vi "AMS Gas cRIO Outer Core.vi"() -> ()   [LabVIEW 2015]
uses:
  Actors/cRIO-CO2/Debugger.ctl
  Actors/cRIO-CO2 Messages/Assign Debugger to Actor Msg/Assign Debugger to Actor Msg.lvclass/Assign Debugger to Actor Msg.ctl
  <vilib>/ActorFramework/Message Enqueuer/Message Enqueuer.lvclass/Message Enqueuer.ctl
  Actors/cRIO-CO2 Messages/Unregister Actor Msg/Unregister Actor Msg.lvclass/Unregister Actor Msg.ctl
  <vilib>/ActorFramework/Message Enqueuer/Enqueue.vi
  <vilib>/ActorFramework/Message Priority Queue/Priority Enqueue.vi
  Actors/cRIO-CO2 Messages/Assign Debugger to Actor Msg/Assign Debugger to Actor Msg.lvclass
  Actors/cRIO-CO2 Messages/Stop All Actors Msg/Stop All Actors Msg.lvclass
  Actors/cRIO-CO2 Messages/Unregister Actor Msg/Unregister Actor Msg.lvclass
  <vilib>/NI_Real-Time Target Support.lvlib
  Actors/cRIO-CO2/cRIO-CO2.lvclass
  <resource>/objmgr/nisysapi.rc
panel:
  out "error out":errorcluster
  in  "Debug":u16(ring)
  out "Debugger Graph Chart":T1(graph)
  in  "Log":i32(listbox)
  out "Thermocouples":T2(graph)
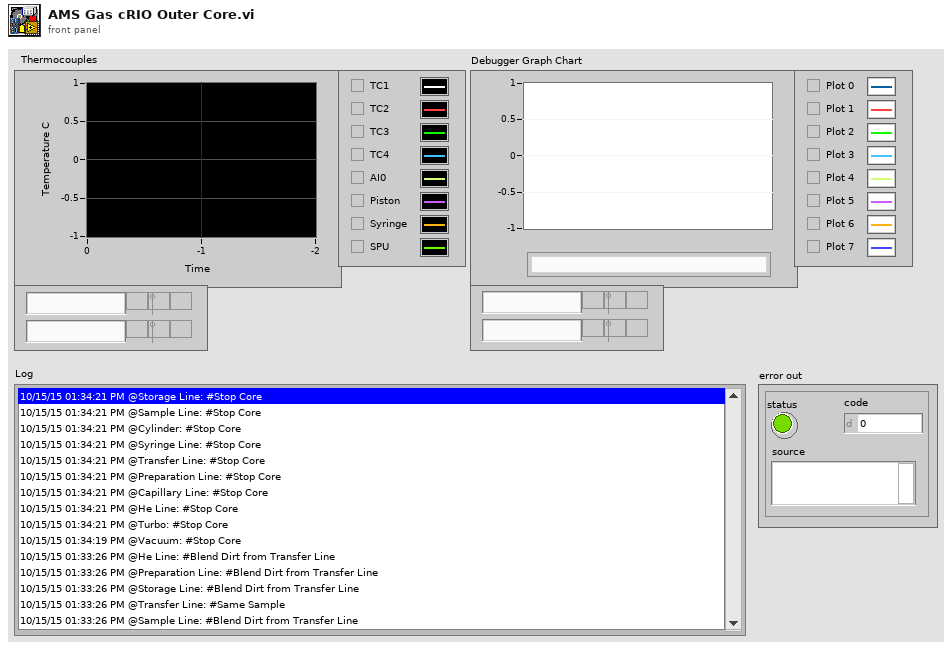
[diagram p1: front panel]
types:
  T1 = cluster{"dT/dt-Lower":dbl, "dT/dt":dbl, "dT/dt 2":dbl, "dT/dt 3":dbl, "dT/dt 4":dbl, "dT/dt-Lower 2":dbl, "dT/dt-Lower 3":dbl, "dT/dt 5":dbl}
  T2 = cluster{dbl, dbl, dbl, dbl, dbl, dbl, dbl, "Total (%)":dbl}
  T3 = cluster{"Numeric 0":dbl, "Numeric 1":dbl, "Numeric 2":dbl, "Numeric 3":dbl, "Numeric 4":dbl, "Numeric 5":dbl, "Numeric 6":dbl, "Numeric 7":dbl}
  T4 = typedef "cRIO-Carbondioxide.lvlib/cRIO-CO2.lvlib/cRIO-CO2.lvclass/Debugger.ctl" = cluster{"Log Ref":refnum<vi>, "Debugger Graph Chart Ref":refnum<vi>, "Debug Rng Ref":refnum<vi>}
  T5 = typedef "NI_Real-Time Target Support.lvlib/RT CPU Load.ctl" = cluster{"Total (%)":dbl, "Time Critical (%)":dbl, "Timed Structures (%)":dbl, "High (%)":dbl, "Above Normal (%)":dbl, "Normal (%)":dbl, "Background (%)":dbl, "Idle (%)":dbl, "ISR (%)":dbl}
  T6 = cluster{"Double":dbl, dbl, dbl, dbl, dbl, dbl, dbl, "Total (%)":dbl}
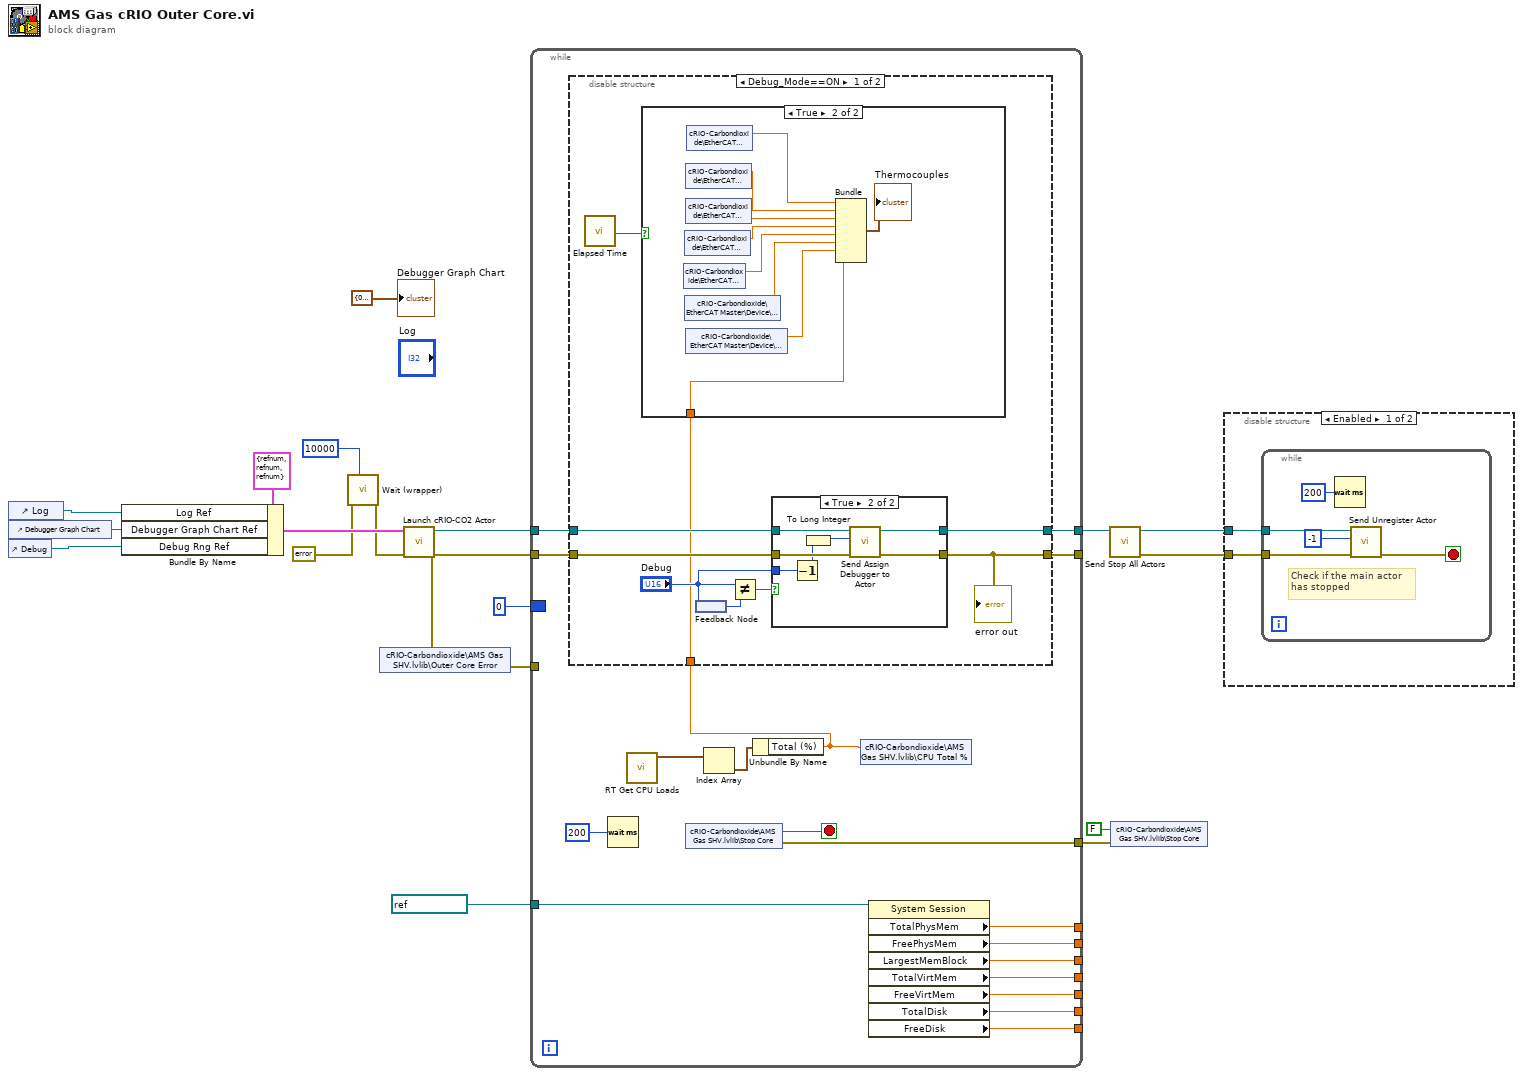
[diagram p0: block diagram]
diagram:
  n1 = control-ref of="Log"() -> (w8:refnum<vi>)
  n2 = control-ref of="Debugger Graph Chart"() -> (w6:refnum<vi>)
  n3 = control-ref of="Debug"() -> (w7:refnum<vi>)
  n4 = Bundle By Name(cluster=T4 {"Log Ref"=refnum, "Debugger Graph Chart Ref"=refnum, "Debug Rng Ref"=refnum} ("Refs for Debuging"), "Log Ref"=w8, "Debugger Graph Chart Ref"=w6, "Debug Rng Ref"=w7) -> (w17:T4)
  n5 = call "Wait (wrapper).vi"("milliseconds to wait (200)"=u32 10000, "error in (no error)"=errorcluster {"status"=FALSE, "code"=0, "source"=""}) -> ("error out"=w4:errorcluster)  [unwired: 9 in]
  n6 = call "Launch cRIO-CO2 Actor.vi"("error in (no error)"=w4, "Refs for Debuging"=w17) -> ("error out"=w11:errorcluster, "Caller-To-Actor Enqueuer"=w19:refnum<class "Message Enqueuer.lvclass">)  [unwired: 8 in]
  n7 = shared-variable "cRIO-Carbondioxide\\AMS Gas SHV.lvlib\\Outer Core Error"(w11) -> (error out=w2:errorcluster)  [unwired: 1 in]
  n8 = while {
    tunnel: w19 -> [w33]
    tunnel: w11 -> [w37]
    tunnel: [w36] -> w16
    border: u16 0 ("Debug") -> [_]
    tunnel: [w35] -> _
    tunnel: [w31] -> w10
    tunnel: w2 -> [_]
    tunnel: refnum<k21> "localhost" ("System Configuration") -> [w27]
    tunnel: [w26] -> _
    tunnel: [w25] -> _
    tunnel: [w24] -> _
    tunnel: [w23] -> _
    tunnel: [w22] -> _
    tunnel: [w21] -> _
    tunnel: [w20] -> _
    stop <- w32 stop-if-true
    n9 = Wait (ms)(milliseconds to wait=u32 200) -> ()  [unwired: 1 out]
    n10 = call <vilib>:"RT Get CPU Loads.vi"() -> ("CPU loads"=w29:T5[])  [unwired: 10 in, 1 out]
    n11 = shared-variable "cRIO-Carbondioxide\\AMS Gas SHV.lvlib\\Stop Core"() -> (w32:bool, error out=w31:errorcluster)  [unwired: 1 in]
    n12 = Index Array(array=w29) -> (element=w30:T5)  [unwired: 1 in]
    n13 = Unbundle By Name(w30) -> ("Total (%)"=w28:dbl)
    n14 = disable-structure shown="Debug_Mode==ON" {
      disable-tunnel: w37 -> [w43 w65]
      disable-tunnel: [w42 w66] -> w36
      disable-tunnel: [w41 w65] -> w35
      disable-tunnel: w33 -> [w39 w66]
      disable-tunnel: w28 -> [w38 _]
      frame condition #0 (active) {
        n15 = call "Elapsed Time"() -> ("Time has Elapsed"=w40:bool)  [unwired: 12 in, 7 out]
        n16 = case shown="True" w40 {
          tunnel: w38 -> [_ w47]
          frame False {
          }
          frame True {
            n17 = shared-variable "cRIO-Carbondioxide\\EtherCAT Master\\Device\\Mod2\\AI0"() -> (w50:dbl)  [unwired: 1 in, 1 out]
            n18 = shared-variable "cRIO-Carbondioxide\\EtherCAT Master\\Device\\Mod1 Storage Line Cold Tank TC 1-4\\TC4"() -> (w51:dbl)  [unwired: 1 in, 1 out]
            n19 = shared-variable "cRIO-Carbondioxide\\EtherCAT Master\\Device\\Mod2\\Piston TC"() -> (w49:dbl)  [unwired: 1 in, 1 out]
            n20 = shared-variable "cRIO-Carbondioxide\\EtherCAT Master\\Device\\Mod1 Storage Line Cold Tank TC 1-4\\TC2"() -> (w53:dbl)  [unwired: 1 in, 1 out]
            n21 = shared-variable "cRIO-Carbondioxide\\EtherCAT Master\\Device\\Mod1 Storage Line Cold Tank TC 1-4\\TC3"() -> (w52:dbl)  [unwired: 1 in, 1 out]
            n22 = shared-variable "cRIO-Carbondioxide\\EtherCAT Master\\Device\\Mod2\\Syringe TC"() -> (w48:dbl)  [unwired: 1 in, 1 out]
            n23 = shared-variable "cRIO-Carbondioxide\\EtherCAT Master\\Device\\Mod1 Storage Line Cold Tank TC 1-4\\TC1"() -> (w55:dbl)  [unwired: 1 in, 1 out]
            n24 = Bundle("Double"=w55, w53, w52, w51, w50, w49, w48, "Total (%)"=w47) -> (→"Thermocouples":T6)  [unwired: 1 in]
          }
        }
        n25 = feedback #1() -> (w46:u16)
        n26 = feedback-in #1("Debug") -> ()
        n27 = Not Equal?(x="Debug", y=w46) -> (x != y?=w45:bool)
        n28 = case shown="True" w45 {
          tunnel: w39 -> [w57 w64]
          tunnel: "Debug" -> [_ w62]
          tunnel: w43 -> [w56 w63]
          tunnel: [w57 w59] -> w42
          tunnel: [w56 w58] -> w41
          frame False {
          }
          frame True {
            n29 = Decrement(x=w62) -> (x-1=w61:u16)
            n30 = To Long Integer(number=w61) -> (32bit integer=w60:i32)
            n31 = call "Send Assign Debugger to Actor.vi"("error in (no error)"=w63, "Actor index"=w60, "Message Enqueuer"=w64) -> ("error out"=w58:errorcluster, "Message Enqueuer out"=w59:refnum<class "Message Enqueuer.lvclass">)  [unwired: 7 in]
          }
        }
        "error out" <- w41
      }
      frame condition #1 {
      }
    }
    n32 = shared-variable "cRIO-Carbondioxide\\AMS Gas SHV.lvlib\\CPU Total %"(w28) -> ()  [unwired: 1 in, 1 out]
    n33 = property class="System Session"(reference=w27) -> ("TotalPhysMem"=w26:dbl, "FreePhysMem"=w25:dbl, "LargestMemBlock"=w24:dbl, "TotalVirtMem"=w23:dbl, "FreeVirtMem"=w22:dbl, "TotalDisk"=w21:dbl, "FreeDisk"=w20:dbl)  [unwired: 1 in, 2 out]
  }
  n34 = call "Send Stop All Actors.vi"("Message Enqueuer"=w16) -> ("error out"=w12:errorcluster, "Message Enqueuer out"=w13:refnum<class "Message Enqueuer.lvclass">)  [unwired: 9 in]
  n35 = shared-variable "cRIO-Carbondioxide\\AMS Gas SHV.lvlib\\Stop Core"(FALSE ("Stop Core"), error in=w10) -> ()  [unwired: 1 out]
  n36 = disable-structure shown="Enabled" {
    disable-tunnel: w12 -> [w67 _]
    disable-tunnel: w13 -> [w68 _]
    frame Enabled {
      n37 = while {
        tunnel: w67 -> [w71]
        tunnel: w68 -> [w72]
        stop <- w69 stop-if-true
        # "Check if the main actor\nhas stopped"
        n38 = Wait (ms)(milliseconds to wait=u32 200) -> ()  [unwired: 1 out]
        n39 = call "Send Unregister Actor.vi"("error in (no error)"=w71, "Index"=-1 ("Actor index"), "Message Enqueuer"=w72) -> ("error out"=w69:errorcluster)  [unwired: 7 in, 1 out]
      }
    }
    frame Disabled {
    }
  }
  "Debugger Graph Chart" <- T3 {"Numeric 0"=0.0, "Numeric 1"=0.0, "Numeric 2"=0.0, "Numeric 3"=0.0, "Numeric 4"=0.0, "Numeric 5"=0.0, "Numeric 6"=0.0, "Numeric 7"=0.0} ("Debugger Graph Chart")
